vi "createCheckOUTInstances.vi"(8 "error in (no error)":errorcluster, 11 "reference in":refnum<class "Items Controller.lvclass">) -> (0 "error out":errorcluster, 3 "reference out":refnum<class "Items Controller.lvclass">)   [LabVIEW 2016, in "Items Controller.lvclass"]
uses:
  Items Controller.lvclass
  storageSheets.ctl
  APP/checkOUT_class/checkOUT.lvclass
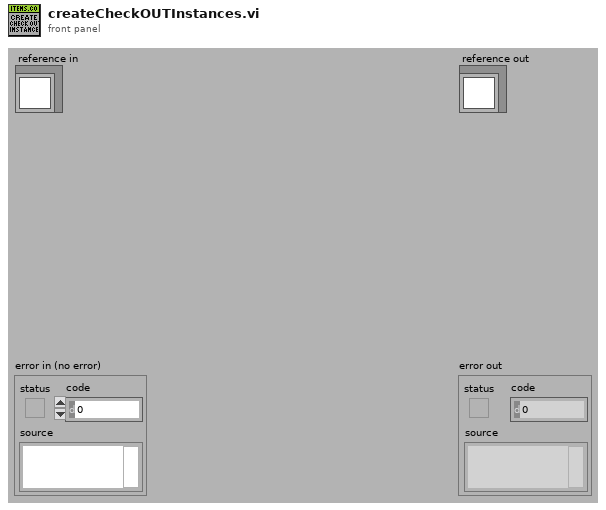
[diagram p1: front panel]
types:
  T1 = typedef "Items Controller.lvclass/storageSheets.ctl" = enum16{"check-in", "check-out", "storage"}
  T2 = typedef "Items Controller.lvclass/ObjectAttributesRef.ctl" = refnum<data-value>
  T3 = typedef "Items Controller.lvclass/ObjectAttributes.ctl" = cluster{"MyAttribute":dbl, "data":string[][][], "file_controller_ref":refnum<class "File Controller.lvclass">, "checkIN_ref":refnum<class "checkIN.lvclass">, "checkOUT_ref":refnum<class "checkOUT.lvclass">, "item_ref":refnum<class "item.lvclass">}
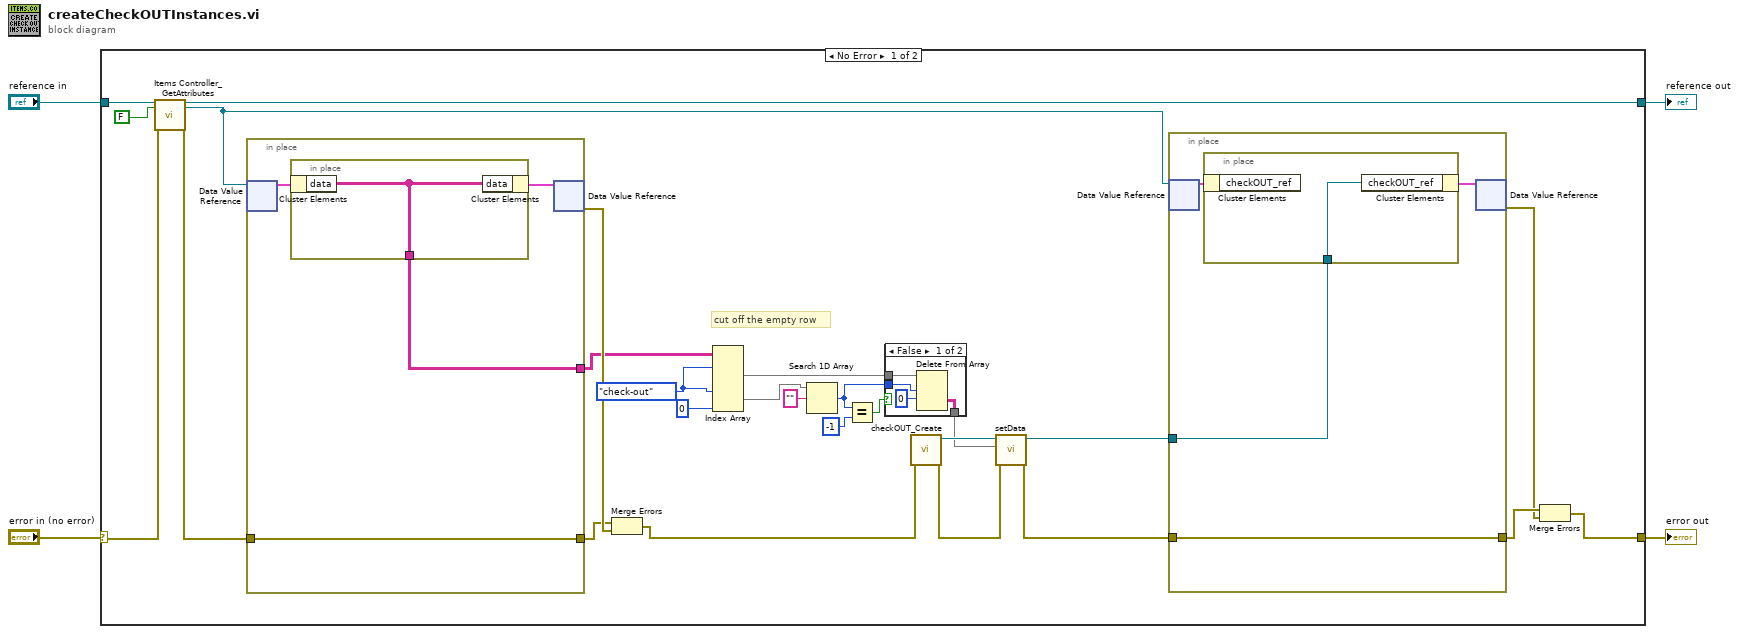
[diagram p0: block diagram]
diagram:
  n1 = case shown="No Error" "error in (no error)" {
    selector: "error in (no error)" -> [w26 w47]
    tunnel: [w20 w47] -> w3
    tunnel: [w24 w46] -> w1
    tunnel: "reference in" -> [w28 w46]
    frame No Error {
      w6 = storageSheets."check-out" ("storageSheets")
      # "cut off the empty row"
      n2 = call "Items Controller_GetAttributes.vi"("reference in"=w28, "return data? (T)"=FALSE, "error in (no error)"=w26) -> ("reference out"=w24:refnum<class "Items Controller.lvclass">, "attributes ref"=w19:T2, "error out"=w25:errorcluster)  [unwired: 13 in, 1 out]
      n3 = in-place {
        in-place-border: w25 -> [w42]
        in-place-border: [w42] -> w29
        in-place-border: [w41] -> w7
        n4 = in-place-dvr #1(w19) -> (w43:T3)  [unwired: 1 out]
        n5 = in-place {
          in-place-border: [w45] -> w41
          n6 = in-place-cluster #2(w43) -> ("data"=w45:string[][][])
          n7 = in-place-cluster #2("data"=w45) -> (w44:T3)
        }
        n8 = in-place-dvr #1(w44) -> (w30:errorcluster)  [unwired: 1 out]
      }
      n9 = Merge Errors(w29, w30) -> (w23:errorcluster)
      n10 = Index Array(array=w7, index (dim 0) #1=w6, index (dim 0) #2=w6, index (dim 2) #2=0 ("disabled index (col)")) -> (element #1=w11:string[][], element #2=w12:string[])  [unwired: 3 in]
      n11 = Search 1D Array(1D array=w12, element="") -> (index of element=w9:i32)  [unwired: 1 in]
      n12 = Equal?(x=w9, y=-1) -> (x = y?=w10:bool)
      n13 = case shown="False" w10 {
        tunnel: w9 -> [w34 _]
        tunnel: w11 -> [w33 w35]
        tunnel: [w31 w35] -> w5
        frame False {
          n14 = Delete From Array(array=w33, length=w34, index (row)=0) -> (deleted portion=w31:string[][])  [unwired: 1 in, 1 out]
        }
        frame True {
        }
      }
      n15 = call "checkOUT_Create.vi"("error in (no error)"=w23) -> ("error out"=w16:errorcluster, "reference out"=w18:refnum<class "checkOUT.lvclass">)  [unwired: 9 in]
      n16 = call "setData.vi"("error in (no error)"=w16, "data"=w5, "reference in"=w18) -> ("error out"=w15:errorcluster, "reference out"=w17:refnum<class "checkOUT.lvclass">)  [unwired: 7 in]
      n17 = in-place {
        in-place-border: w15 -> [w37]
        in-place-border: [w37] -> w22
        in-place-border: w17 -> [w36]
        n18 = in-place-dvr #3(w19) -> (w38:T3)  [unwired: 1 out]
        n19 = in-place {
          in-place-border: w36 -> [w40]
          n20 = in-place-cluster #4(w38) -> ()  [unwired: 1 out]
          n21 = in-place-cluster #4("checkOUT_ref"=w40) -> (w39:T3)
        }
        n22 = in-place-dvr #3(w39) -> (w21:errorcluster)  [unwired: 1 out]
      }
      n23 = Merge Errors(w22, w21) -> (w20:errorcluster)
    }
    frame Error {
    }
  }
  "error out" <- w3
  "reference out" <- w1
